vi "Pre Launch Init.vi"(11 "Nested in":refnum<class "Microscope Controller.lvclass">) -> (0 "error out":errorcluster, 3 "Nested out":refnum<class "Microscope Controller.lvclass">)   [LabVIEW 2020, in "Microscope Controller.lvlib" / "Microscope Controller.lvclass"]
doc: "(<B>Filename</B>: Actor Framework.lvlib:Actor.lvclass:Pre Launch Init.vi)\n\nDefines behavior that occurs after the Launch Nested Actor method is invoked but before the actor's Actor Core method begins running.\n\nBy default, this method does nothing. A descendant class may override it to define behavior."
uses:
  Microscope Controller.lvclass
  Microscope Controller.lvclass/Microscope Controller.ctl
  <vilib>/ActorFramework/Actor/Actor.lvclass
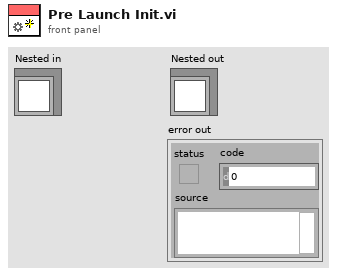
[diagram p1: front panel]
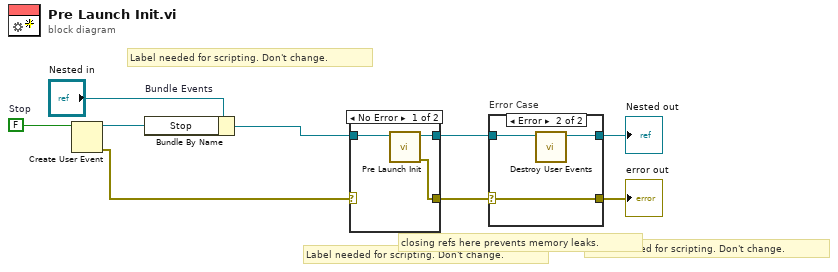
[diagram p0: block diagram]
diagram:
  w8 = FALSE  # Stop
  # "Label needed for scripting. Don't change."
  # "Label needed for scripting. Don't change."
  # "Label needed for scripting. Don't change."
  # "closing refs here prevents memory leaks."
  n1 = Create User Event(user event datatype=w8) -> (user event=w5:refnum<user-event>, error out=w7:errorcluster)  [unwired: 1 in]
  n2 = Bundle By Name "Bundle Events"(cluster="Nested in", "Stop"=w5) -> (w2:refnum<class "Microscope Controller.lvclass">)
  n3 = case shown="No Error" w7 {
    selector: w7 -> [_ w14]
    tunnel: [w12 w13] -> w3
    tunnel: w2 -> [w11 w13]
    tunnel: [w10 w14] -> w1
    frame No Error {
      n4 = call-parent "Pre Launch Init.vi"("Actor in"=w11) -> ("error out"=w10:errorcluster, "Actor out"=w12:refnum<class "Microscope Controller.lvclass">)  [unwired: 9 in]
    }
    frame Error {
    }
  }
  n5 = case "Error Case" shown="Error" w1 {
    selector: w1 -> [w15 w19]
    tunnel: w3 -> [w16 w18]
    tunnel: [w16 w17] -> w6
    tunnel: [w15 w19] -> w4
    frame No Error {
    }
    frame Error {
      n6 = call "Destroy User Events.vi"("UI Template in"=w18) -> ("UI Template out"=w17:refnum<class "Microscope Controller.lvclass">)  [unwired: 10 in]
    }
  }
  "error out" <- w4
  "Nested out" <- w6
